vi "solar_voy_def Items Bit Size.vi"(10 "ITEMS":T1[](array[typedef])) -> (1 "Byte Size":i32, 2 "Bit Size":i32)   [LabVIEW 2018]
doc: "This calculates the total bit size of the items. Note: This does not account for dynamically sized items at the end of the packet."
uses:
  solar_voy_def_ctl ITEM TYPE.ctl
  type/solar_type Item Type.ctl
  solar_voy_def_ctl ITEM.ctl
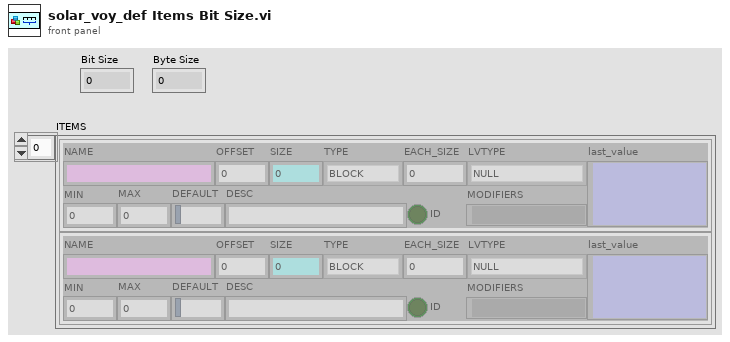
[diagram p1: front panel]
types:
  T1 = typedef "solar_voy_def_ctl ITEM.ctl" = cluster{"NAME":string, "OFFSET":i32, "SIZE":i32, "TYPE":T2, "EACH_SIZE":i32, "LVTYPE":T3, "MIN":dbl, "MAX":dbl, "DEFAULT":string, "DESC":string, "ID":bool, "MODIFIERS":variant, "last_value":variant}
  T2 = typedef "solar_voy_def_ctl ITEM TYPE.ctl" = enum8{"BLOCK", "INT", "UINT", "FLOAT", "STRING"}
  T3 = typedef "solar_type Item Type.ctl" = enum16{"NULL", "UNKNOWN", "CLUSTER", "I8", "I16", "I32", "I64", "U8", "U16", "U32", "U64", "U8_ENUM", "U16_ENUM", "U32_ENUM", "SGL", "DBL", "BOOLEAN", "STRING", "PATH", "VISA", "TAG", "TIME", "I8_1D", "I16_1D", "I32_1D", "I64_1D", "U8_1D", "U16_1D", "U32_1D", "U64_1D", "U8_ENUM_1D", "U16_ENUM_1D", "U32_ENUM_1D", "SGL_1D", "DBL_1D", "BOOLEAN_1D", "STRING_1D", "PATH_1D", "VISA_1D", "TAG_1D", "TIME_1D", "I8_2D", "I16_2D", "I32_2D", "I64_2D", "U8_2D", "U16_2D", "U32_2D", "U64_2D", "U8_ENUM_2D", "U16_ENUM_2D", "U32_ENUM_2D", "SGL_2D", "DBL_2D", "BOOLEAN_2D", "STRING_2D", "PATH_2D", "VISA_2D", "TAG_2D", "TIME_2D"}
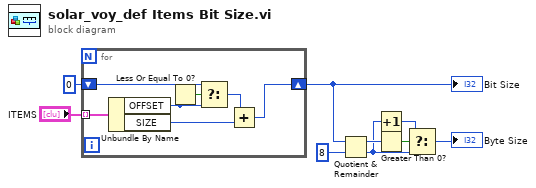
[diagram p0: block diagram]
diagram:
  n1 = for {
    tunnel: "ITEMS" -> [w16] mode=indexing
    shift-right: [w10] -> w7
    shift-left: 0 ("OFFSET") -> [w14]
    n2 = Unbundle By Name(w16) -> ("OFFSET"=w12:i32, "SIZE"=w15:i32)
    n3 = Less Or Equal To 0?(x=w12) -> (x <= 0?=w13:bool)
    n4 = Select(t=w14, s=w13, f=w12) -> (s? t:f=w11:i32)
    n5 = Add(x=w11, y=w15) -> (x+y=w10:i32)
  }
  "Bit Size" <- w7
  n6 = Quotient & Remainder(x=w7, y=8) -> (x-y*floor(x/y)=w5:i32, floor(x/y)=w3:i32)
  n7 = Increment(x=w3) -> (x+1=w2:i32)
  n8 = Greater Than 0?(x=w5) -> (x > 0?=w4:bool)
  n9 = Select(t=w2, s=w4, f=w3) -> (s? t:f=→"Byte Size":i32)
